vi "readLossSpecFromExcel.vi"(8 "错误输入（无错误）":errorcluster, 10 "Spec Points":dbl, 11 "Spec Path":path) -> (0 "错误输出":errorcluster, 3 "lossSpec":string[][](table))   [LabVIEW 2011]
panel:
  in  "Excel._Worksheet":refnum<k7>
  in  "Excel._Application":refnum<k7>
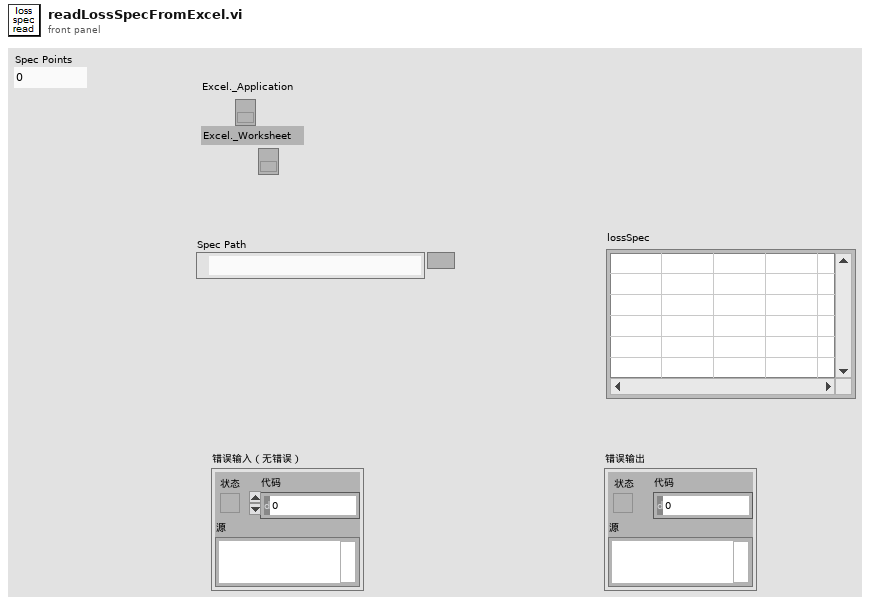
[diagram p1: front panel]
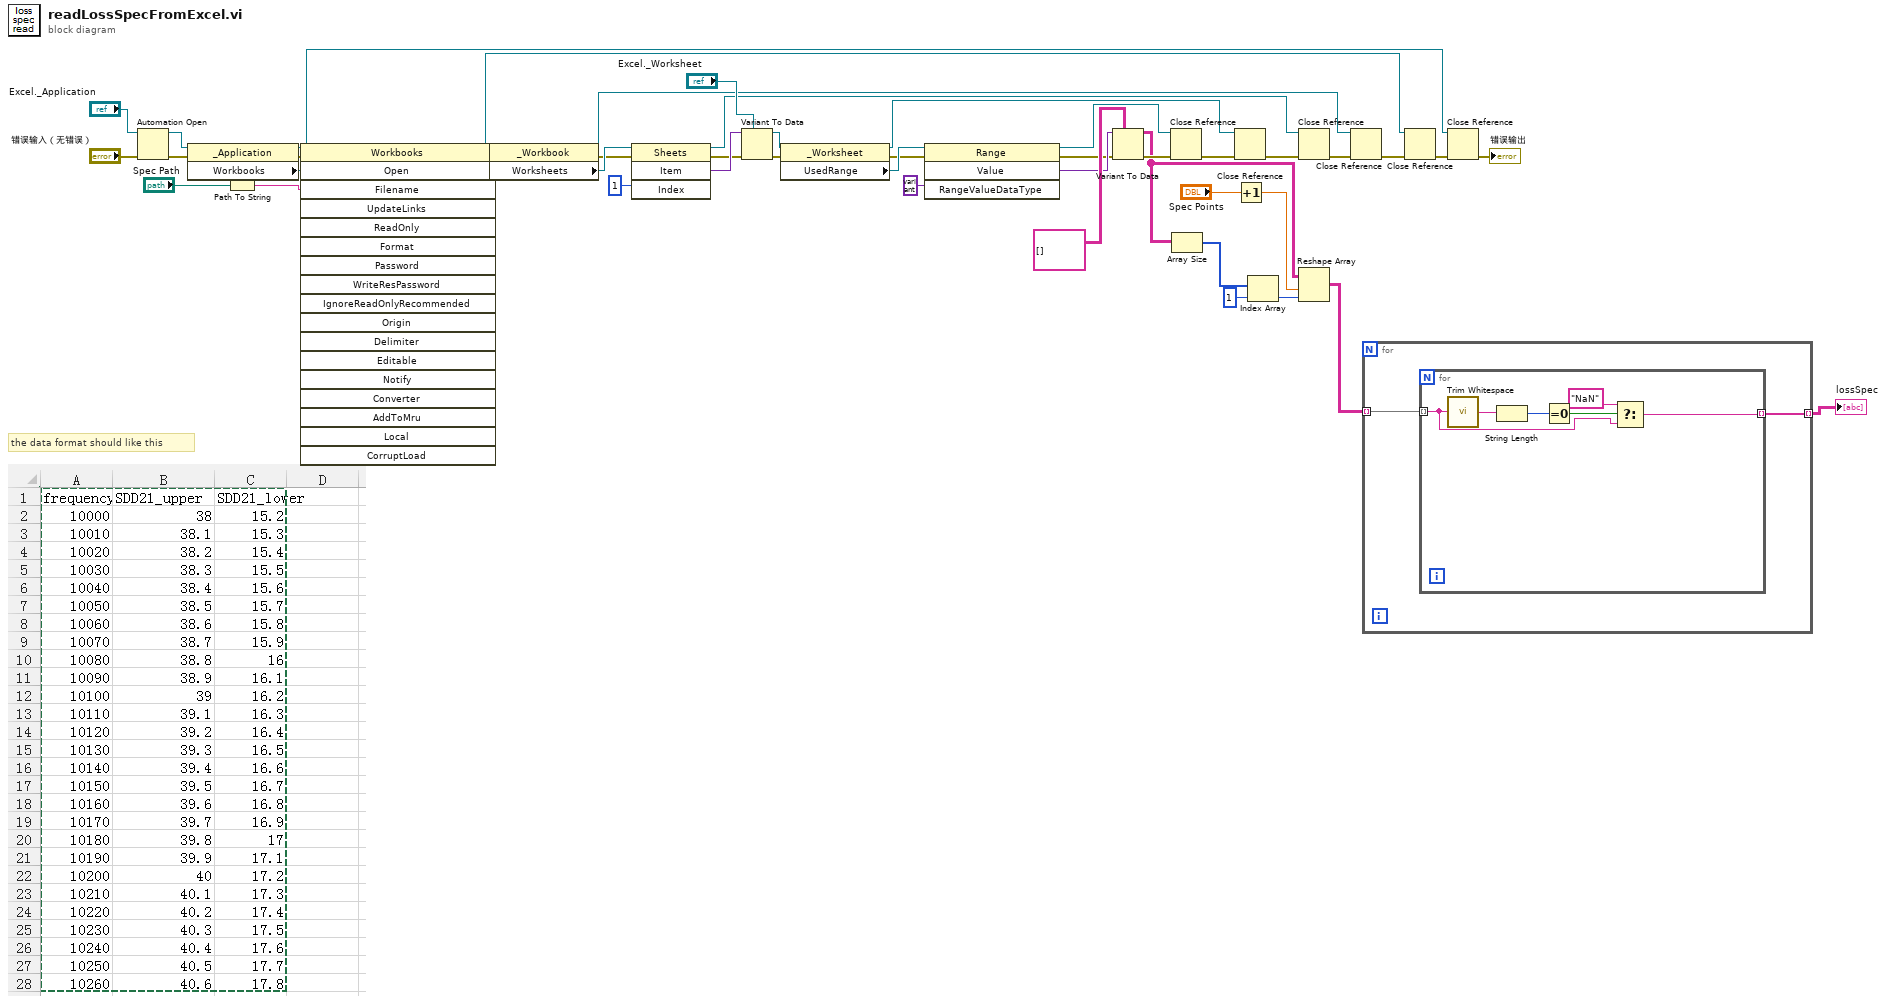
[diagram p0: block diagram]
diagram:
  # "the data format should like this"
  n1 = Automation Open(error in (no error)="错误输入（无错误）", Automation Refnum="Excel._Application") -> (Automation Refnum=w44:refnum<k7>, error out=w29:errorcluster)  [unwired: 2 in]
  n2 = property class="_Application"(reference=w44, error in=w29) -> (reference out=w11:refnum<k7>, error out=w28:errorcluster, "Workbooks"=w43:refnum<k7>)
  n3 = Path To String(path="Spec Path") -> (string=w41:string)
  n4 = invoke class="Workbooks" method="Open"(reference=w43, error in=w28, "Filename"=w41) -> (reference out=w13:refnum<k7>, error out=w27:errorcluster, "Open"=w40:refnum<k7>)  [unwired: 15 in, 15 out]
  n5 = property class="_Workbook"(reference=w40, error in=w27) -> (reference out=w15:refnum<k7>, error out=w26:errorcluster, "Worksheets"=w39:refnum<k7>)
  n6 = invoke class="Sheets" method="Item"(reference=w39, error in=w26, "Index"=1) -> (reference out=w17:refnum<k7>, error out=w25:errorcluster, "Item"=w38:variant)  [unwired: 1 in, 1 out]
  n7 = Variant To Data(error in=w25, type="Excel._Worksheet", Variant=w38) -> (data=w36:refnum<k7>, error out=w24:errorcluster)
  n8 = property class="_Worksheet"(reference=w36, error in=w24) -> (reference out=w19:refnum<k7>, error out=w23:errorcluster, "UsedRange"=w35:refnum<k7>)
  n9 = invoke class="Range" method="Value"(reference=w35, error in=w23, "RangeValueDataType"=variant) -> (reference out=w21:refnum<k7>, error out=w22:errorcluster, "Value"=w32:variant)  [unwired: 1 in, 1 out]
  n10 = Variant To Data(error in=w22, type=string[][] [] ("添加的数组"), Variant=w32) -> (data=w8:string[][], error out=w20:errorcluster)
  n11 = Close Reference(reference=w21, error in (no error)=w20) -> (error out=w18:errorcluster)
  n12 = Array Size(array=w8) -> (size(s)=w5:i32[])
  n13 = Close Reference(reference=w19, error in (no error)=w18) -> (error out=w16:errorcluster)
  n14 = Increment(x="Spec Points") -> (x+1=w6:dbl)
  n15 = Index Array(array=w5, index=1 ("索引")) -> (element=w3:i32)
  n16 = Close Reference(reference=w17, error in (no error)=w16) -> (error out=w14:errorcluster)
  n17 = Reshape Array(w8, w6, w3) -> (w2:string[][])
  n18 = Close Reference(reference=w15, error in (no error)=w14) -> (error out=w12:errorcluster)
  n19 = for {
    tunnel: w2 -> [w47] mode=indexing
    tunnel: [w46] -> w1 mode=indexing
    n20 = for {
      tunnel: w47 -> [w49] mode=indexing
      tunnel: [w48] -> w46 mode=indexing
      n21 = call <vilib>:"Trim Whitespace.vi"("string"=w49) -> ("trimmed string"=w53:string)  [unwired: 1 in]
      n22 = String Length(string=w53) -> (length=w52:i32)
      n23 = Equal To 0?(x=w52) -> (x = 0?=w51:bool)
      n24 = Select(t="NaN", s=w51, f=w49) -> (s? t:f=w48:string)
    }
  }
  "lossSpec" <- w1
  n25 = Close Reference(reference=w13, error in (no error)=w12) -> (error out=w10:errorcluster)
  n26 = Close Reference(reference=w11, error in (no error)=w10) -> (error out=→"错误输出":errorcluster)
